vi "Export Frames Properties.vi"(8 "error in (no error)":errorcluster, 10 "PID Inputs GUID":string, 11 "Section Ref out in":T1 format="%.0x") -> (0 "error out":errorcluster, 2 "Frames Array":T2[](array[typedef]) {"Signals"."Byte Order" items=["Little Endian", "Big Endian"]; "Signals"."Data Type" items=["Signed", "Unsigned", "IEEE Float"]}, 3 "Section Ref out":T1 format="%.0x")   [LabVIEW 2015, in "Diagnostics Addon System Explorer.lvlib"]
uses:
  System Explorer/Diagnostics Addon System Explorer.lvlib
  <vilib>/NI Veristand/Custom Device API/Custom Device Item Ref.ctl
  Frame Parameters.ctl
  Signal Parameters.ctl
  ID FG.vi
  Get Signals.vi
  Signal Parameters FG.vi
  <vilib>/NI Veristand/Custom Device API/NI VeriStand - Get Custom Device Channel Data.vi
  <vilib>/NI Veristand/Custom Device API/NI VeriStand - Get Item Description.vi
  <vilib>/NI Veristand/Custom Device API/NI VeriStand - Get Item Property.vi
  <vilib>/NI Veristand/Custom Device API/Get Item Property (String).vi
  <vilib>/NI Veristand/Custom Device API/Get Item Property (Double).vi
  <vilib>/NI Veristand/Custom Device API/Get Item Property (U32).vi
  <vilib>/NI Veristand/Custom Device API/NI VeriStand - Set Item Property.vi
  <vilib>/NI Veristand/Custom Device API/Set Item Property (String).vi
  <vilib>/NI Veristand/Custom Device API/Set Item Property (Double).vi
  <vilib>/NI Veristand/Custom Device API/Set Item Property (U32).vi
  GUID Lookup.vi
  <vilib>/NI Veristand/Custom Device API/NI VeriStand - Get Item Data.vi
  <vilib>/NI Veristand/Custom Device Tools/Custom Device Utility Library/NI VeriStand - Search for Item by GUID.vi
  <vilib>/NI Veristand/Custom Device Tools/Custom Device Utility Library/Custom Device Utility Library.lvlib
  <vilib>/NI Veristand/Custom Device API/Custom Device API.lvlib
  Diagnostics Addon Shared.lvlib
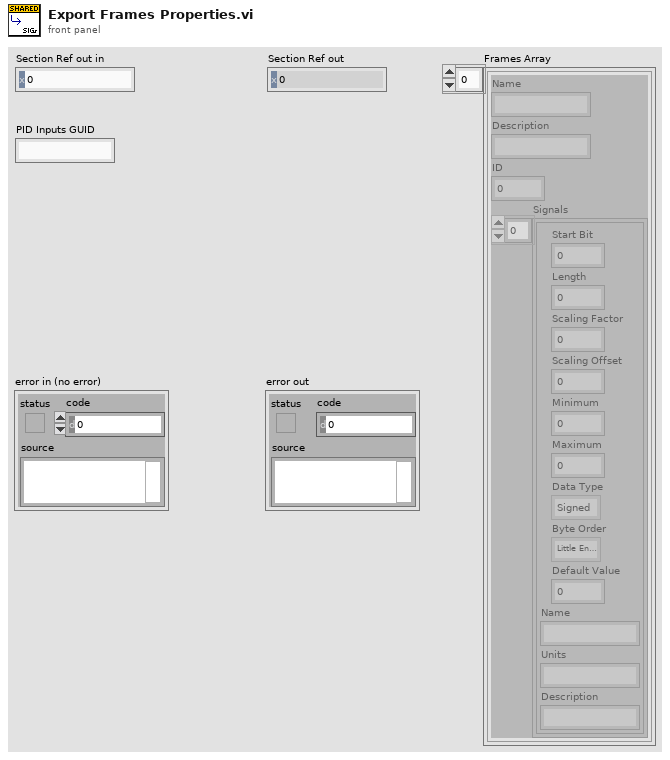
[diagram p1: front panel]
types:
  T1 = typedef "Custom Device API.lvlib/Custom Device Item Ref.ctl" = u64
  T2 = typedef "Diagnostics Addon Shared.lvlib/Frame Parameters.ctl" = cluster{"Name":string, "Description":string, "ID":u16, "Signals":T3[]}
  T3 = typedef "Diagnostics Addon Shared.lvlib/Signal Parameters.ctl" = cluster{"Start Bit":u8, "Length":u8, "Scaling Factor":dbl, "Scaling Offset":dbl, "Minimum":dbl, "Maximum":dbl, "Data Type":u32, "Byte Order":u32, "Default Value":dbl, "Name":string, "Units":string, "Description":string}
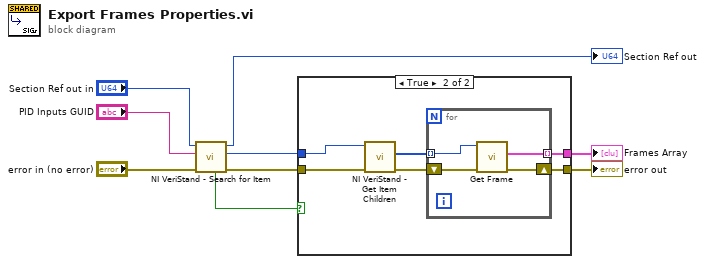
[diagram p0: block diagram]
diagram:
  n1 = call-poly <vilib>:"NI VeriStand - Search for Item.vi"("error in"="error in (no error)", "Item GUID"="PID Inputs GUID", "Section Ref in"="Section Ref out in") -> ("error out"=w5:errorcluster, "Item Ref"=w6:T1, "Section Ref out"=→"Section Ref out":T1, "Found"=w1:bool)  [unwired: 5 in]
  n2 = case shown="True" w1 {
    tunnel: [w10 w16] -> w8
    tunnel: [_ w15] -> w7
    tunnel: w6 -> [_ w13]
    tunnel: w5 -> [w10 w11]
    frame False {
    }
    frame True {
      n3 = call <vilib>:"NI VeriStand - Get Item Children.vi"("error in (no error)"=w11, "Item Ref in"=w13) -> ("error out"=w12:errorcluster, "Child Refs"=w14:T1[])  [unwired: 6 in, 2 out]
      n4 = for {
        shift-right: [w19] -> w16
        shift-left: w12 -> [w20]
        tunnel: w14 -> [w18] mode=indexing
        tunnel: [w17] -> w15 mode=indexing
        n5 = call "Get Frame.vi"("error in (no error)"=w20, "Item Ref in"=w18) -> ("error out"=w19:errorcluster, "PID In"=w17:T2)  [unwired: 7 in, 1 out]
      }
    }
  }
  "error out" <- w8
  "Frames Array" <- w7
